vi "Check Output For Octave Errors.vi"(8 "error in":errorcluster, 10 "read buffer":string) -> (0 "error out":errorcluster)   [LabVIEW 2020, in "GOLPI library.lvlib"]
doc: "Parse stdout output of GNU Octave and search for GNU Octave errors. If any found, generates LabVIEW error.\n\n---\nGOLPI works only with lv_pro.dll library, which is part of vipm package or should be delivered together with packed library. Placement of this dll is selected in terminal of Start GNU Octave.vi."
uses:
  GOLPI library.lvlib
  Custom Error Codes Enum Type Def.vi
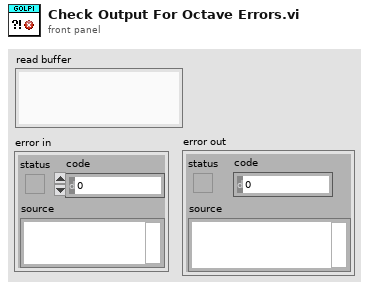
[diagram p1: front panel]
types:
  T1 = typedef "GOLPI library.lvlib/Custom Error Codes Enum Type Def.vi" = enum16{"no error", "00 working directory PAR1 missing", "01 octave binary PAR1 missing", "02 octave report error PAR1", "03 empty output last cmd PAR1", "04 missing temporary file PAR1", "05 pwd PAR 1 not exist", "06 oct package not installed", "07 octave default binary missing", "10 var PAR1 not string, vect", "11 var PAR1 not num, scal, ~compl", "12 var PAR1 not num, scal, compl", "13 var PAR1 not num, vect, ~compl", "14 var PAR1 not num, vect, compl", "15 var PAR1 not num, mat, ~compl", "16 var PAR1 not num, mat, ~compl", "30 read timeout", "60 bitstream transport failed", "61 bitstream decode error PAR1", "62 bitstream cannot be set", "70 struct transfer not possible", "80 struct: cluster elem. PAR1 not implem.", "81 struct: structure field PAR1 not implem.", "82 struct: size mismatch of PAR1", "83 struct: type mismatch of PAR1", "98 internal error", "99 not finished", "90 Not supported in Matlab mode", "91 Matlab variable transfer error", "92 Matlab Script Error"}
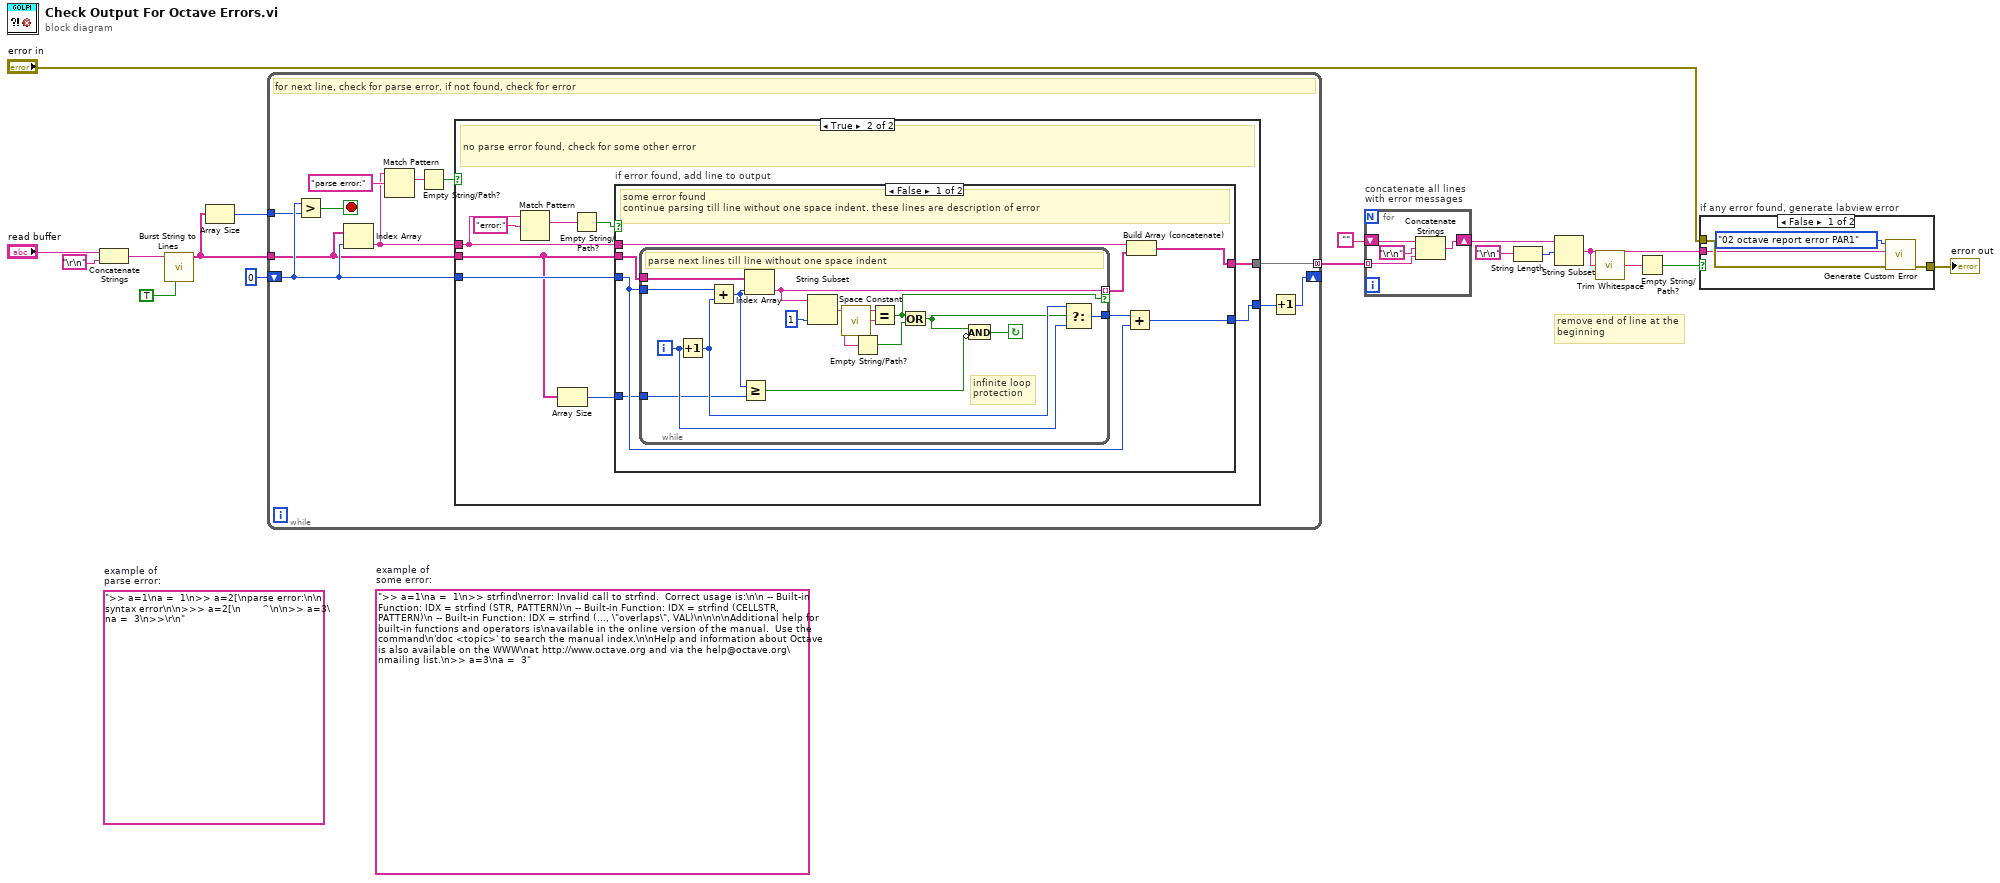
[diagram p0: block diagram]
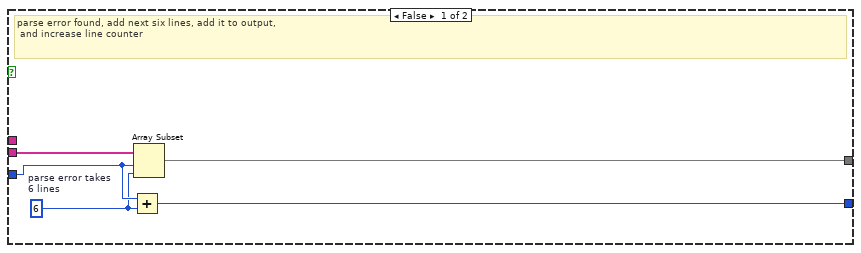
[diagram p2: hidden frame]
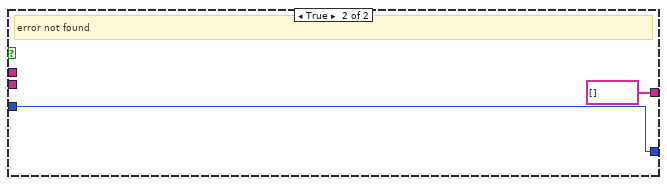
[diagram p3: hidden frame]
diagram:
  (unwired) ">> a=1\na =  1\n>> strfind\nerror: Invalid call to strfind.  Correct usage is:\n\n -- Built-in Function: IDX = strfind (STR, PATTERN)\n -- Built-in Function: IDX = strfind (CELLSTR, PATTERN)\n -- Built-in Function: IDX = strfind (..., \"overlaps\", VAL)\n\n\n\nAdditional help for built-in functions and operators is\navailable in the online version of the manual.  Use the command\n'doc <topic>' to search the manual index.\n\nHelp and information about Octave is also available on the WWW\nat http://www.octave.org and via the help@octave.org\nmailing list.\n>> a=3\na =  3"  # example of some error:
  (unwired) ">> a=1\na =  1\n>> a=2[\nparse error:\n\n  syntax error\n\n>>> a=2[\n       ^\n\n>> a=3\na =  3\n>>\r\n"  # example of parse error:
  # "remove end of line at the\nbeginning"
  n1 = Concatenate Strings("read buffer", "\r\n") -> (w3:string)
  n2 = call "Burst String to Lines.vi"("preserve leading spaces"=TRUE, "read buffer"=w3) -> ("lines"=w2:string[])  [unwired: 9 in]
  n3 = Array Size(array=w2) -> (size(s)=w8:i32)
  n4 = while {
    shift-right: [w20] -> _
    shift-left: 0 ("index") -> [w24]
    tunnel: [w25] -> w10 mode=concatenating
    tunnel: w8 -> [w23]
    tunnel: w2 -> [w19]
    stop <- w22 stop-if-true
    # "for next line, check for parse error, if not found, check for error"
    n5 = Greater?(x=w24, y=w23) -> (0:w22:bool)
    n6 = Index Array(array=w19, index=w24) -> (element=w18:string)
    n7 = Match Pattern(string=w18, regular expression="parse error:") -> (match substring=w27:string)  [unwired: 1 in, 3 out]
    n8 = Empty String/Path?(string/path=w27) -> (empty?=w26:bool)
    n9 = case shown="True" w26 {
      tunnel: w19 -> [w32 w35]
      tunnel: w24 -> [w31 w37]
      tunnel: [w29 w39] -> w25
      tunnel: [w33 w36] -> w21
      tunnel: w18 -> [_ w38]
      frame False {
        w30 = 6  # parse error takes 6 lines
        # "parse error found, add next six lines, add it to output,\n and increase line counter"
        n10 = Add(x=w31, y=w30) -> (x+y=w33:i32)
        n11 = Array Subset(array=w32, index=w31, length=w30) -> (w29:string[])
      }
      frame True {
        # "no parse error found, check for some other error"
        n12 = Match Pattern(string=w38, regular expression="error:") -> (match substring=w42:string)  [unwired: 1 in, 3 out]
        n13 = Array Size(array=w35) -> (size(s)=w34:i32)
        n14 = Empty String/Path?(string/path=w42) -> (empty?=w40:bool)
        n15 = case "if error found, add line to output" shown="False" w40 {
          tunnel: [w49 string[] []] -> w39
          tunnel: w38 -> [w50 _]
          tunnel: w35 -> [w48 _]
          tunnel: w37 -> [w45 w67]
          tunnel: [w44 w67] -> w36
          tunnel: w34 -> [w43 _]
          frame False {
            # "some error found\ncontinue parsing till line without one space indent. these lines are description of error"
            n16 = while {
              tunnel: w48 -> [w66]
              tunnel: w45 -> [w65]
              tunnel: [w60] -> w47 mode=indexing if=w56
              tunnel: [w57] -> w46
              tunnel: w43 -> [w51]
              i -> [w58]
              stop <- w55 continue-if-true
              # "infinite loop\nprotection"
              # "parse next lines till line without one space indent"
              n17 = Increment(x=w58) -> (x+1=w59:i32)
              n18 = Add(x=w65, y=w59) -> (x+y=w52:i32)
              n19 = Greater Or Equal?(x=w52, y=w51) -> (x >= y?=w53:bool)
              n20 = Index Array(array=w66, index=w52) -> (element=w60:string)
              n21 = String Subset(string=w60, length (rest)=1 ("length (rest)")) -> (substring=w62:string)  [unwired: 1 in]
              n22 = call <vilib>:"Space Constant.vi"() -> ("String"=w63:string)
              n23 = Empty String/Path?(string/path=w62) -> (empty?=w61:bool)
              n24 = Equal?(x=w62, y=w63) -> (x = y?=w56:bool)
              n25 = Or(x=w56, y=w61) -> (x .or. y?=w54:bool)
              n26 = Compound Arithmetic op=AND(w54, invert w53) -> (w55:bool)
              n27 = Select(t=w59, s=w54, f=w58) -> (s? t:f=w57:i32)
            }
            n28 = Add(x=w46, y=w45) -> (x+y=w44:i32)
            n29 = Build Array (concatenate)(w50, w47) -> (w49:string[])
          }
          frame True {
            # "error not found"
          }
        }
      }
    }
    n30 = Increment(x=w21) -> (x+1=w20:i32)
  }
  n31 = for "concatenate all lines\nwith error messages" {
    tunnel: w10 -> [w70] mode=indexing
    shift-right: [w72] -> w7
    shift-left: "" -> [w69]
    n32 = Concatenate Strings(w69, "\r\n", w70) -> (w72:string)
  }
  n33 = String Length(string="\r\n") -> (length=w4:i32)
  n34 = String Subset(string=w7, offset (0)=w4) -> (substring=w6:string)  [unwired: 1 in]
  n35 = call <vilib>:"Trim Whitespace.vi"("string"=w6) -> ("trimmed string"=w12:string)  [unwired: 1 in]
  n36 = Empty String/Path?(string/path=w12) -> (empty?=w17:bool)
  n37 = case "if any error found, generate labview error" shown="False" w17 {
    tunnel: w6 -> [w73 _]
    tunnel: "error in" -> [w76 w77]
    tunnel: [w75 w77] -> w15
    frame False {
      n38 = call "Generate Custom Error.vi"("error in"=w76, "PAR1"=w73, "GOLPI error"=Custom_Error_Codes_Enum_Type_Def.vi."02 octave report error PAR1" ("Enum")) -> ("error out"=w75:errorcluster)  [unwired: 8 in]
    }
    frame True {
    }
  }
  "error out" <- w15
